vi "OBIS Laser State.vi"() -> ()   [LabVIEW 8.6]
uses:
  <vilib>/Instr/_visa.llb/VISA Configure Serial Port (Instr).vi
panel:
  out "On/Off":string
  out "Mode":string
  in  "Set/Query?":bool caption="Set / Query?"
  in  "Operating Mode":u16(ring) items=["CW Constant Power", "CW Constant Current", "Pulsed Digital", "Pulsed Analog", "Pulsed Mixed"]
  in  "Laser On/Off":bool
  in  "VISA resource name":refnum<visa-resource-name>
  # "Set"
  # "Query"
  # "This VI can be used to turn the laser emission on or off and can be used to select the operational mode of the laser.  The VI can be set to either just query those settings or to set them into the laser.  Select the appropriate VISA resouce name (COM port number) for the laser and whether to set or query and then run the VI."
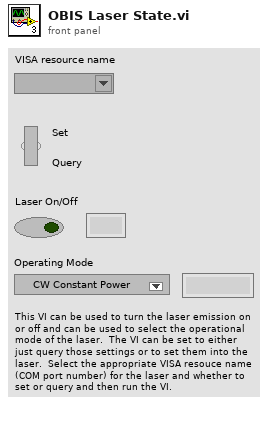
[diagram p1: front panel]
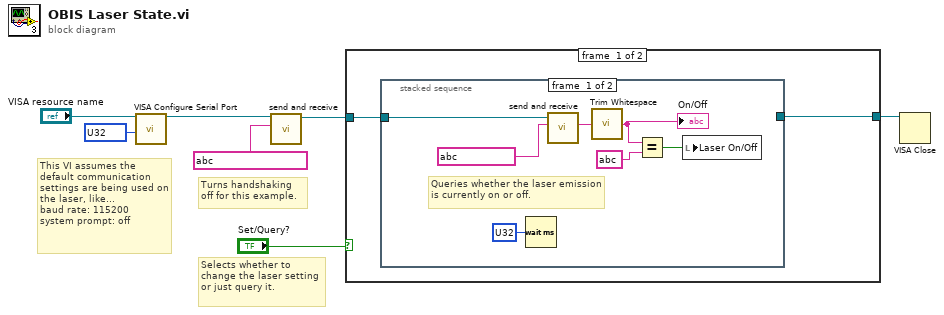
[diagram p0: block diagram]
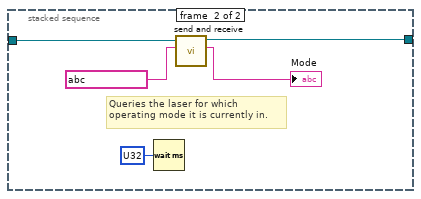
[diagram p2: hidden frame]
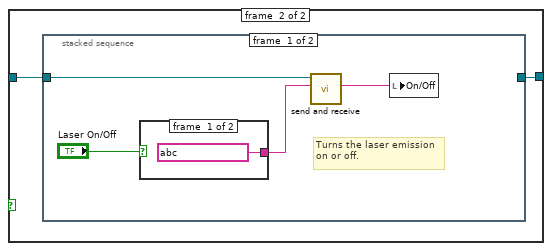
[diagram p3: hidden frame]
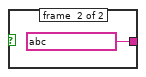
[diagram p4: hidden frame]
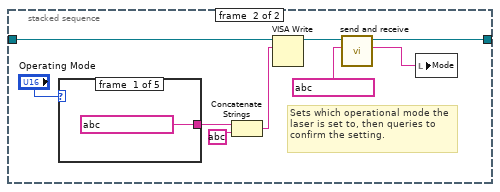
[diagram p5: hidden frame]
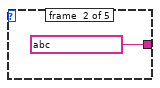
[diagram p6: hidden frame]
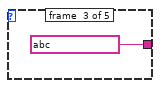
[diagram p7: hidden frame]
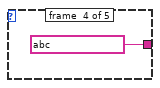
[diagram p8: hidden frame]
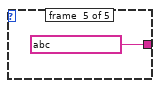
[diagram p9: hidden frame]
diagram:
  # "Selects whether to change the laser setting or just query it."
  # "Turns handshaking\noff for this example."
  # "This VI assumes the default communication settings are being used on the laser, like...\nbaud rate: 115200\nsystem prompt: off"
  n1 = call-poly "VISA Configure Serial Port"("VISA resource name"="VISA resource name", "baud rate (9600)"=u32 ?) -> ("VISA resource name out"=w4:refnum<visa-resource-name>)  [unwired: 12 in, 1 out]
  n2 = call "send and receive.vi"("write to laser"=string ?, "VISA resource name"=w4) -> ("VISA resource name out"=w3:refnum<visa-resource-name>)  [unwired: 8 in, 1 out]
  n3 = case shown="True" "Set/Query?" {
    tunnel: w3 -> [w9 w23]
    tunnel: [w8 w22] -> w1
    frame #0 {
      n4 = stacked-sequence {
        tunnel: w9 -> [w14 w19]
        tunnel: [_ w18] -> w8
        frame #0 {
          # "Queries whether the laser emission is currently on or off."
          n5 = Wait (ms)(milliseconds to wait=u32 ?) -> ()  [unwired: 1 out]
          n6 = call "send and receive.vi"("write to laser"=string ?, "VISA resource name"=w14) -> ("read from laser"=w12:string)  [unwired: 8 in, 1 out]
          n7 = call <vilib>:"Trim Whitespace.vi"("string"=w12) -> ("trimmed string"=w10:string)  [unwired: 1 in]
          "On/Off" <- w10
          n8 = Equal?(x=w10, y=string ?) -> (x = y?=w11:bool)
          n9 = local write "Laser On/Off"(w11) -> ()
        }
        frame #1 {
          # "Queries the laser for which operating mode it is currently in."
          n10 = Wait (ms)(milliseconds to wait=u32 ?) -> ()  [unwired: 1 out]
          n11 = call "send and receive.vi"("write to laser"=string ?, "VISA resource name"=w19) -> ("read from laser"=→"Mode":string, "VISA resource name out"=w18:refnum<visa-resource-name>)  [unwired: 8 in]
        }
      }
    }
    frame #1 {
      n12 = stacked-sequence {
        tunnel: w23 -> [w26 w35]
        tunnel: [_ w31] -> w22
        frame #0 {
          # "Turns the laser emission on or off."
          n13 = case shown="True" "Laser On/Off" {
            tunnel: [string ? string ?] -> w25
            frame #0 {
            }
            frame #1 {
            }
          }
          n14 = call "send and receive.vi"("write to laser"=w25, "VISA resource name"=w26) -> ("read from laser"=w24:string)  [unwired: 8 in, 1 out]
          n15 = local write "On/Off"(w24) -> ()
        }
        frame #1 {
          # "Sets which operational mode the laser is set to, then queries to confirm the setting."
          n16 = case shown="2" "Operating Mode" {
            tunnel: [string ? string ? string ? string ? string ?] -> w36
            frame #0 {
            }
            frame #1 {
            }
            frame #2 {
            }
            frame #3 {
            }
            frame #4 {
            }
          }
          n17 = Concatenate Strings(w36, string ?) -> (w38:string)
          n18 = VISA Write(VISA resource name=w35, write buffer=w38) -> (VISA resource name out=w33:refnum<visa-resource-name>)  [unwired: 1 in, 2 out]
          n19 = call "send and receive.vi"("write to laser"=string ?, "VISA resource name"=w33) -> ("read from laser"=w32:string, "VISA resource name out"=w31:refnum<visa-resource-name>)  [unwired: 8 in]
          n20 = local write "Mode"(w32) -> ()
        }
      }
    }
  }
  n21 = VISA Close(VISA resource name=w1) -> ()  [unwired: 1 in, 1 out]
